vi "FGPA Main.vi"() -> ()   [LabVIEW 2014]
doc: "This is the main FPGA VI for the SPI application. It sets up the SPI communication and then runs the SPI engine. In a parallel loop, data is continually read from the Real Time application and sent to the SPI engine. The SPI engine handles all communication between the FPGA and the SPI chip."
uses:
  <userlib>/_NI SPI IP/FPGA/Controllers/Public/Transfer Settings.ctl
  <vilib>/Platform/TimedLoop/XDataNode/timing_clust.ctl
  <vilib>/Platform/TimedLoop/XDataNode/nitl_modes.ctl
  <vilib>/Platform/TimedLoop/XDataNode/wakeup.ctl
  vi.lib/SPIAPI/DIO/SPI Digital IO Lines.ctl
  <vilib>/rvi/Emulation/niFpgaGetClockAttributes.vi
  <vilib>/rvi/Emulation/niFpgaSctlEmulationGetInTimedLoop.vi
  <vilib>/rvi/Emulation/niFpgaEmulationReportErrorSimple.vi
  <vilib>/rvi/Emulation/niFpgaCriticalErrorInLSC.vi
  <vilib>/Platform/TimedLoop/XDataNode/XDataNode.xnode
  <vilib>/Platform/TimedLoop/XDataNode/XDNodeRunTimeDep.lvlib
  <userlib>/_NI SPI IP/FPGA/Controllers/NI SPI IP FPGA.lvlib
panel:
  out "Response from Slave":u64
  out "read Iterations":i32
  in  "Data To Slave":u64=2147483648
  in  "Chip Select":u8
  in  "SPI PHY Settings":T1={"Divide Value"=20, "Transfer Length (bits)"=32, "CS Asserted Polarity"=FALSE, "Clock Polarity (CPOL)"=FALSE, "Clock Phase (CPHA)"=FALSE, "Lengthen MISO Setup"=FALSE, "Direction Change Bit"=0, "MOSI Starts as Output"=FALSE, "Tristatable MOSI"=FALSE} {"Direction Change Bit" max=64 step=1; "Transfer Length (bits)" min=1 max=64 step=1}
  in  "Data Rate (S/s)":u32=10000
  out "oclk freq":u32
  out "oclk div":u32
  out "FPGA Error":errorcluster
  out "Acq Loop Ticks":u32
  # "Overview: This is the FPGA VI that communicates with the MAX5216.\nRequirements: LabVIEW Full Development System, LabVIEW Real Time,  LabVIEW FPGA, MAX5216, NI System on Module, NI 9651.\nInstructions:\nRun RT Main without making adjustments to this VI to avoid a recompile.  If you desire to adjust this VI, do so, \nthen be sure to point RT Main to this VI instead of the pre-compiled bitfile that it currently targets."
  # "OUTPUT"
  # "INPUT"
  # "ADC Data::Debug"
  # "Acquisition Parameters"
  # "SPI PHY Settings"
  # "Debug"
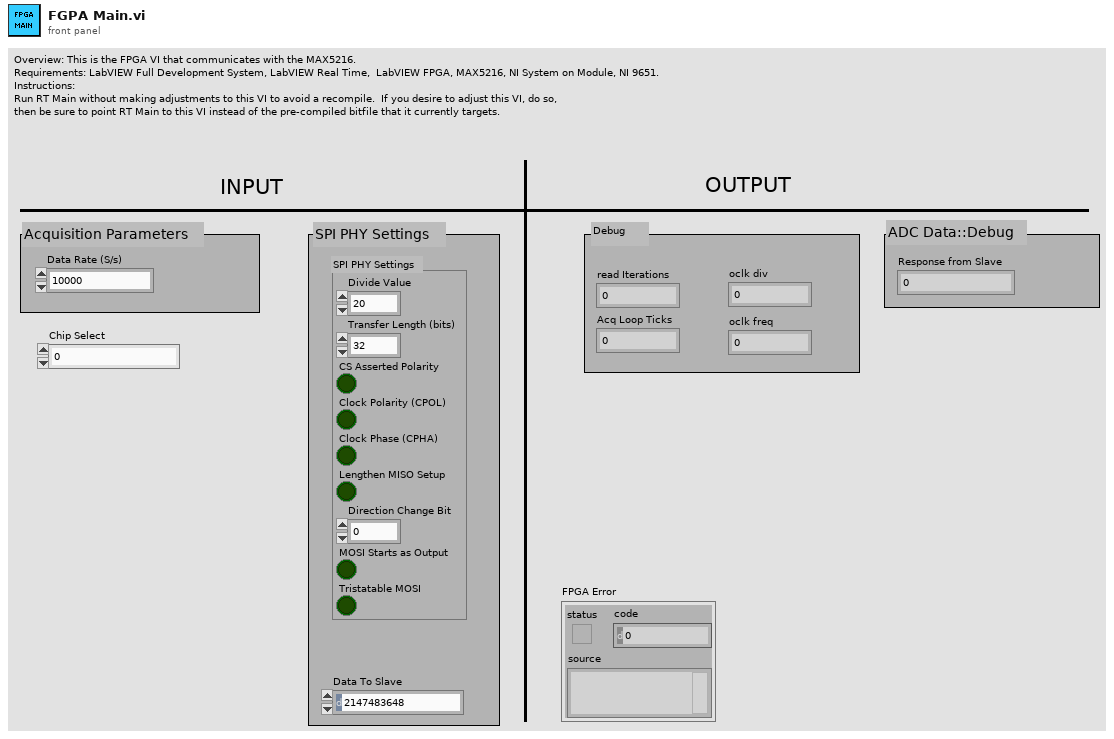
[diagram p1: front panel]
types:
  T1 = typedef "NI SPI IP FPGA.lvlib/Transfer Settings.ctl" = cluster{"Divide Value":u8, "Transfer Length (bits)":u8, "CS Asserted Polarity":bool, "Clock Polarity (CPOL)":bool, "Clock Phase (CPHA)":bool, "Lengthen MISO Setup":bool, "Direction Change Bit":u8, "MOSI Starts as Output":bool, "Tristatable MOSI":bool}
  T2 = typedef "SPI Digital IO Lines.ctl" = cluster{"SCLK":refnum<k21>, "MISO":refnum<k21>, "MOSI":refnum<k21>, "CS 0":refnum<k21>, "CS 1":refnum<k21>, "CS 2":refnum<k21>, "CS 3":refnum<k21>, "CS 4":refnum<k21>, "CS 5":refnum<k21>}
  T3 = typedef "Internal Data (SPI API).ctl" = cluster{"DLU To SPI Engine Data FIFO":refnum<k21>, "SPI Engine to DLU Data FIFO":refnum<k21>, "Data to SPI Engine (Cache) Register":refnum<k21>, "SPI PHY Settings to SPI Engine (Cahche) Register":refnum<k21>}
  T4 = typedef "XDNodeRunTimeDep.lvlib/timing_clust.ctl" = cluster{"Expected End [f-1]":u64, "Actual End [f-1]":u64, "Finished Late? [f-1]":bool, "Expected End [i-1]":u64, "Actual End [i-1]":u64, "Finished Late? [i-1]":bool, "Expected Start [i]":u64, "Actual Start [i]":u64, "Expected Start [f]":u64, "Actual Start [f]":u64, "Source Name":string, "Structure Name":string, "Period":i64, "Deadline":i64, "Offset":i64, "Start":i64, "Priority":i32, "Timeout":i32, "Mode":T5, "Wakeup Reason":T6, "Error":errorcluster, "Source Type":string, "Secondary Source Type":string, "Global End Time":u64, "Global Start Time":u64, "Frame Duration":u64, "Iteration Duration":u64, "Assigned CPU":i32, "I/O Scan Engine Mode":u32}
  T5 = typedef "XDNodeRunTimeDep.lvlib/nitl_modes.ctl" = enum32{"No Change", "Process missed periods, maintain original phase", "Discard missed periods, maintain original phase", "Process missed periods, ignore original phase", "Discard missed periods, ignore original phase"}
  T6 = typedef "XDNodeRunTimeDep.lvlib/wakeup.ctl" = enum32{"Normal", "Aborted", "Asynchronous wakeup", "Timing source error", "Timed loop error", "Timeout"}
  T7 = typedef "SPI Response Information.ctl" = cluster{"Data to Node":u64, "Node Id":u16}
  T8 = typedef "NI SPI IP FPGA.lvlib/Spi Master Inputs.ctl" = cluster{"MISO":bool}
  T9 = typedef "NI SPI IP FPGA.lvlib/Spi Master Outputs.ctl" = cluster{"Chip Select":bool, "Clock":bool, "MOSI":bool, "MOSI OE":bool}
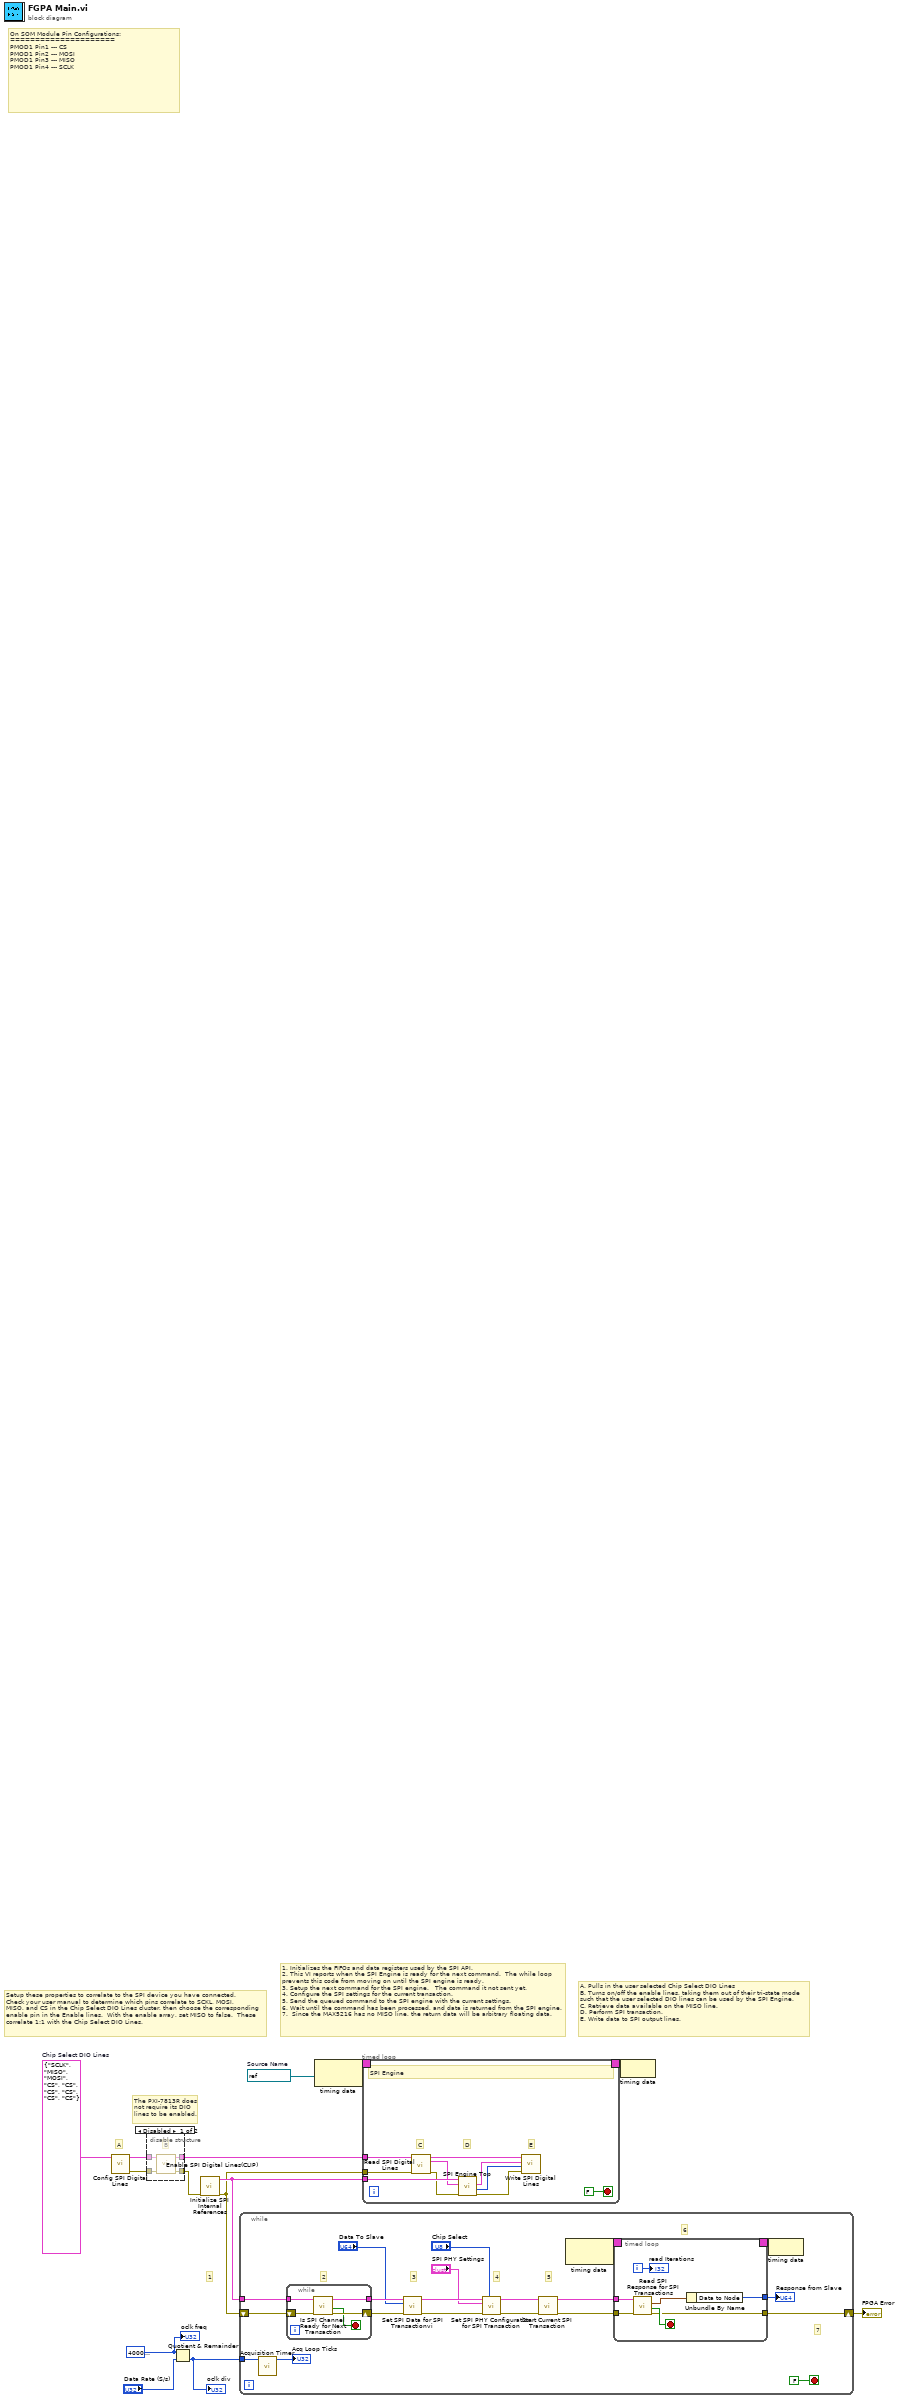
[diagram p0: block diagram]
diagram:
  w5 = T2 {"SCLK"="SCLK", "MISO"="MISO", "MOSI"="MOSI", "CS 0"="CS", "CS 1"="CS", "CS 2"="CS", "CS 3"="CS", "CS 4"="CS", "CS 5"="CS"}  # Chip Select DIO Lines
  w9 = refnum<k21> "120MHz"  # Source Name
  w11 = u32 40000000 ("oclk freq")
  # "The PXI-7813R does\nnot require its DIO \nlines to be enabled."
  # "A. Pulls in the user selected Chip Select DIO Lines\nB. Turns on/off the enable lines, taking them out of their tri-state mode \nsuch that the user selected DIO lines can be used by the SPI Engine.\nC. Retrieve data available on the MISO line.\nD. Perform SPI transaction.\nE. Write data to SPI output lines."
  # "A"
  # "1. Initializes the FIFOs and data registers used by the SPI API.\n2. This VI reports when the SPI Engine is ready for the next command.  The while loop \nprevents this code from moving on until the SPI engine is ready.\n3. Setup the next command for the SPI engine.   The command it not sent yet.\n4. Configure the SPI settings for the current transaction.\n5. Send the queued command to the SPI engine with the current settings.\n6. Wait until the command has been processed, and data is returned from the SPI engine.\n7.  Since the MAX5216 has no MISO line, the return data will be arbitrary floating data."
  # "1"
  # "Setup these properties to correlate to the SPI device you have connected.\nCheck your user manual to determine which pins correlate to SCKL, MOSI,\nMISO, and CS in the Chip Select DIO Lines cluster, then choose the corresponding\nenable pin in the Enable lines.  With the enable array, set MISO to false.  These\ncorrelate 1:1 with the Chip Select DIO Lines."
  # "On SOM Module Pin Configurations:\n=====================\nPMOD1 Pin1 --- CS\nPMOD1 Pin2 --- MOSI\nPMOD1 Pin3 --- MISO\nPMOD1 Pin4 --- SCLK"
  n1 = call "Config SPI Digital Lines.vi"("SPI DIO Lines"=w5) -> ("error out"=w6:errorcluster, "Chip Select DIO Lines"=w7:T2)  [unwired: 9 in]
  n2 = disable-structure shown="Disabled" {
    disable-tunnel: [w18 w20] -> w8
    disable-tunnel: [w17 w19] -> w2
    disable-tunnel: w7 -> [w16 w20]
    disable-tunnel: w6 -> [w15 w19]
    frame Disabled {
      # "B"
      n3 = call "Enable SPI Digital Lines(CLIP).vi"("error in"=w15, "SPI DIO Lines"=w16) -> ("error out"=w17:errorcluster, "Chip Select DIO Lines"=w18:T2)  [unwired: 8 in]
    }
    frame Enabled {
    }
  }
  n4 = Quotient & Remainder(x=w11, y="Data Rate (S/s)") -> (floor(x/y)=w1:u32)  [unwired: 1 out]
  "oclk div" <- w1
  n5 = call "Initialize SPI Internal References.vi"("error in"=w2) -> ("error out"=w3:errorcluster, "SPI API References"=w10:T3)  [unwired: 9 in]
  n6 = while {
    tunnel: w1 -> [w40]
    shift-right: [w24] -> w4
    shift-left: w3 -> [w35]
    tunnel: w10 -> [w36]
    stop <- FALSE stop-if-true
    # "7"
    # "6"
    # "5"
    # "4"
    # "3"
    # "2"
    n7 = call <vilib>:"Acquisition Timer.vi"("Loop Time (Ticks)"=w40) -> ("Actual Time (Ticks)"=→"Acq Loop Ticks":u32)  [unwired: 10 in]
    n8 = while {
      shift-right: [w45] -> w38
      shift-left: w35 -> [w42]
      tunnel: w36 -> [w43]
      tunnel: [w44] -> w37
      stop <- w41 stop-if-true
      n9 = call "Is SPI Channel Ready for Next Transaction.vi"("error in"=w42, "Private Data In"=w43) -> ("error out"=w45:errorcluster, "SPI Channel Ready"=w41:bool, "Private Data Out"=w44:T3)  [unwired: 6 in, 1 out]
    }
    n10 = call "Set SPI Data for SPI Transactionvi.vi"("error in"=w38, "Data In"="Data To Slave", "Private Data In"=w37) -> ("error out"=w30:errorcluster, "Private Data Out"=w31:T3)  [unwired: 7 in]
    n11 = call "Set SPI PHY Configuration for SPI Transaction.vi"("Chip Select"="Chip Select", "error in"=w30, "SPI PHY Settings"="SPI PHY Settings", "Private Data In"=w31) -> ("error out"=w27:errorcluster, "Private Data Out"=w28:T3)  [unwired: 6 in]
    n12 = call "Start Current SPI Transaction.vi"("error in"=w27, "Private Data In"=w28) -> ("error out"=w32:errorcluster, "Private Data Out"=w26:T3)  [unwired: 7 in, 1 out]
    n13 = node-c288() -> (w34:T4)  [unwired: 1 in]
    n14 = timed-loop {
      timing: w34 -> [_]
      timing-out: [_] -> w33
      tunnel: w32 -> [w52]
      tunnel: w26 -> [w51]
      tunnel: [w46] -> w23
      tunnel: [w48] -> w24
      i -> [w47]
      stop <- w50 stop-if-true
      n15 = call "Read SPI Response for SPI Transactions.vi"("error in"=w52, "Private Data In"=w51) -> ("error out"=w48:errorcluster, "Read Data Valid?"=w50:bool, "Read Data"=w49:T7)  [unwired: 6 in, 1 out]
      n16 = Unbundle By Name(w49) -> ("Data to Node"=w46:u64)
      "read Iterations" <- w47
    }
    "Response from Slave" <- w23
    n17 = node-c288(w33) -> ()
  }
  "FPGA Error" <- w4
  n18 = node-c288(w9) -> (w14:T4)
  n19 = timed-loop {
    tunnel: w10 -> [w64]
    tunnel: w3 -> [w62]
    tunnel: w8 -> [w65]
    timing: w14 -> [_]
    timing-out: [_] -> w13
    stop <- FALSE stop-if-true
    # "E"
    # "D"
    # "C"
    # "SPI Engine"
    n20 = call "Read SPI Digital Lines.vi"("Chip Select DIO Lines"=w65, "error in"=w62) -> ("Chip Select DIO Lines Out"=w66:T2, "SPI Read Data"=w63:T8, "error out"=w61:errorcluster)  [unwired: 11 in]
    n21 = call "SPI Engine Top.vi"("error in"=w61, "SPI Read Data"=w63, "SPI API References"=w64) -> ("error out"=w60:errorcluster, "Chip Select ID"=w59:u8, "SPI DIO Output"=w58:T9)  [unwired: 5 in, 1 out]
    n22 = call "Write SPI Digital Lines.vi"("error in"=w60, "CS Index"=w59, "spi output"=w58, "Chip Select DIO Lines"=w66) -> ()  [unwired: 6 in, 2 out]
  }
  n23 = node-c288(w13) -> ()
  "oclk freq" <- w11
